vi "Errors.vi"   [LabVIEW 2017, in "DSF Core.lvlib" / "Thread Parameters.lvclass"]
uses:
  Thread Parameters.lvclass
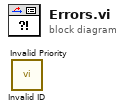
[diagram p0: block diagram]
diagram:
  n1 = call "Invalid ID.vi"() -> ()  [unwired: 10 in, 2 out]
  n2 = call "Invalid Priority.vi"() -> ()  [unwired: 10 in, 2 out]
